vi "closeConnection.vi"(8 "error in (no error)":errorcluster, 11 "RaspberryPi in":refnum<class "RaspberryPi.lvclass">) -> (0 "error out":errorcluster, 3 "RaspberryPi out":refnum<class "RaspberryPi.lvclass">)   [LabVIEW 2020, in "RaspberryPi.lvclass"]
uses:
  RaspberryPi.lvclass
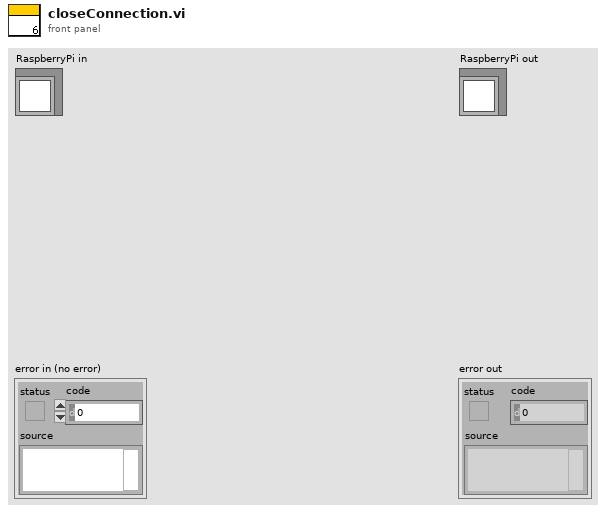
[diagram p1: front panel]
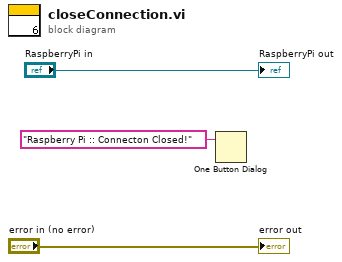
[diagram p0: block diagram]
diagram:
  n1 = One Button Dialog(message="Raspberry Pi :: Connecton Closed!") -> ()  [unwired: 1 in, 1 out]
  "error out" <- "error in (no error)"
  "RaspberryPi out" <- "RaspberryPi in"
